vi "Eval X-Y(t) Optimal Step.vi"(4 "number of points":u32=10, 5 "Formulas":string[](array[string])=["  ", "  "], 6 "end":dbl=1.0 format="%.2f", 7 "start":dbl format="%.2f", 8 "epsilon":dbl=0.05 min=1e-18 format="%.2f") -> (0 "error":i32, 1 "ticks":u32, 2 "Y":dbl[](array[numeric]) format="%.2f", 3 "X":dbl[](array[numeric]) format="%.2f")   [LabVIEW 2017, in "NI_Gmath.lvlib"]
doc: "Calculates the values of a more complex function (f(t),g(t)), where t runs over an interval. Both components are given by <B>Formulas</B>."
uses:
  NI_Gmath.lvlib
panel:
  # "Example:\n\n number of points: 100\n epsilon: 0.05 \n start: 0.0\n end: 1.0\n Formulas: sin(t*t)+t and exp(-t)"
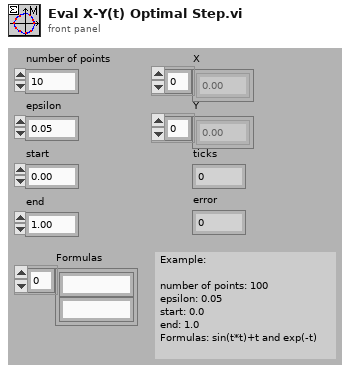
[diagram p1: front panel]
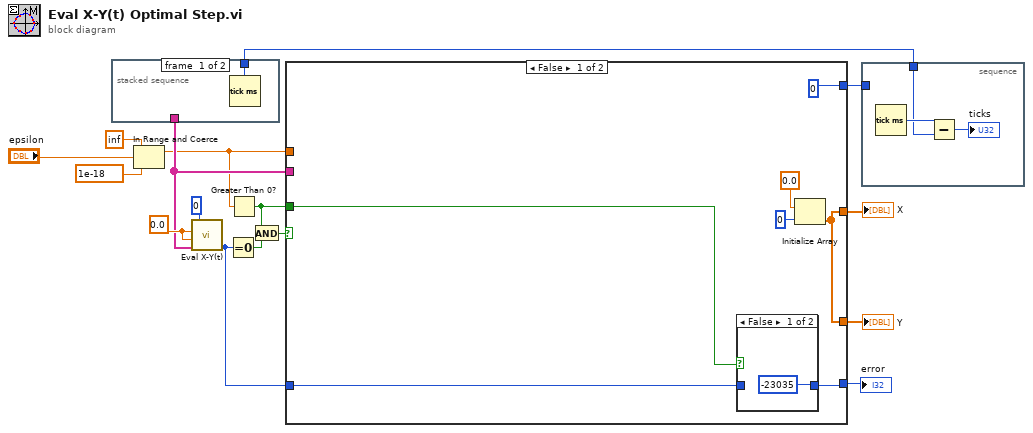
[diagram p0: block diagram]
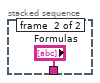
[diagram p2: hidden frame]
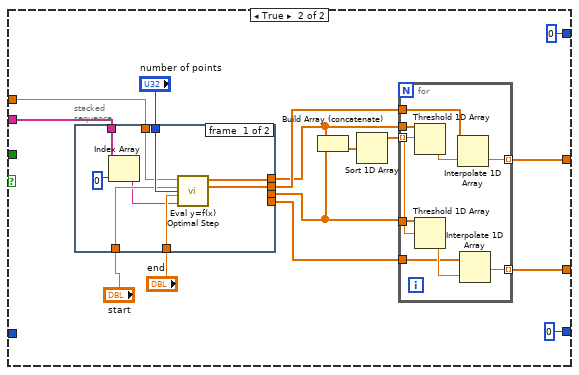
[diagram p4: hidden frame]
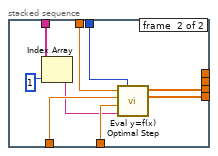
[diagram p5: hidden frame]
diagram:
  w11 = 0.0
  n1 = stacked-sequence {
    tunnel: [w17 _] -> w16
    tunnel: [_ "Formulas"] -> w5
    frame #0 {
      n2 = Tick Count (ms)() -> (millisecond timer value=w17:u32)
    }
    frame #1 {
    }
  }
  n3 = In Range and Coerce(upper limit=inf, x="epsilon", lower limit=1e-18) -> (coerced(x)=w1:dbl)  [unwired: 1 out]
  n4 = call "Eval X-Y(t).vi"("Formulas"=w5, "end"=w11, "start"=w11, "number of points"=u32 0) -> ("error"=w6:i32)  [unwired: 3 out]
  n5 = Equal To 0?(x=w6) -> (x = 0?=w10:bool)
  n6 = Greater Than 0?(x=w1) -> (x > 0?=w7:bool)
  n7 = And(x=w7, y=w10) -> (x .and. y?=w9:bool)
  n8 = case shown="False" w9 {
    tunnel: [w22 w31] -> w14
    tunnel: [0 0] -> w15
    tunnel: [w22 w32] -> w13
    tunnel: w5 -> [_ w30]
    tunnel: w1 -> [_ w29]
    tunnel: [w19 0] -> w8
    tunnel: w7 -> [w21 _]
    tunnel: w6 -> [w20 _]
    frame False {
      n9 = case shown="False" w21 {
        tunnel: w20 -> [_ w27]
        tunnel: [-23035 w27] -> w19
        frame False {
        }
        frame True {
        }
      }
      n10 = Initialize Array(0.0, 0) -> (w22:dbl[])
    }
    frame True {
      n11 = stacked-sequence {
        tunnel: w30 -> [w51 w60]
        tunnel: "number of points" -> [w47 w56]
        tunnel: w29 -> [w46 w55]
        tunnel: "end" -> [w44 w53]
        tunnel: "start" -> [w45 w54]
        tunnel: [w49 _] -> w33
        tunnel: [_ w58] -> w42
        tunnel: [_ w57] -> w38
        tunnel: [w48 _] -> w41
        frame #0 {
          n12 = Index Array(array=w51, index=0) -> (element=w43:string)
          n13 = call "Eval y=f(x) Optimal Step.vi"("number of points"=w47, "formula"=w43, "end"=w44, "start"=w45, "epsilon"=w46) -> ("Y Values"=w48:dbl[], "X Values"=w49:dbl[])  [unwired: 2 out]
        }
        frame #1 {
          n14 = Index Array(array=w60, index=1) -> (element=w52:string)
          n15 = call "Eval y=f(x) Optimal Step.vi"("number of points"=w56, "formula"=w52, "end"=w53, "start"=w54, "epsilon"=w55) -> ("Y Values"=w57:dbl[], "X Values"=w58:dbl[])  [unwired: 2 out]
        }
      }
      n16 = Build Array (concatenate)(w33, w42) -> (w39:dbl[])
      n17 = Sort 1D Array(array=w39) -> (sorted array=w40:dbl[])
      n18 = for {
        tunnel: w33 -> [w69]
        tunnel: w40 -> [w61] mode=indexing
        tunnel: w41 -> [w67]
        tunnel: [w66] -> w31 mode=indexing
        tunnel: w42 -> [w65]
        tunnel: w38 -> [w63]
        tunnel: [w62] -> w32 mode=indexing
        n19 = Threshold 1D Array(2:w61, 3:w69) -> (0:w68:dbl)  [unwired: 1 in]
        n20 = Threshold 1D Array(2:w61, 3:w65) -> (0:w64:dbl)  [unwired: 1 in]
        n21 = Interpolate 1D Array(1:w68, 2:w67) -> (0:w66:dbl)
        n22 = Interpolate 1D Array(1:w64, 2:w63) -> (0:w62:dbl)
      }
    }
  }
  "X" <- w14
  "Y" <- w13
  "error" <- w8
  n23 = stacked-sequence {
    tunnel: w16 -> [w70]
    tunnel: w15 -> [_]
    frame #0 {
      n24 = Tick Count (ms)() -> (millisecond timer value=w71:u32)
      n25 = Subtract(x=w71, y=w70) -> (x-y=→"ticks":u32)
    }
  }
